vi "例4.3.vi"() -> ()   [LabVIEW 2018]
panel:
  out "MAX":dbl
  in  "y":dbl
  in  "x":dbl
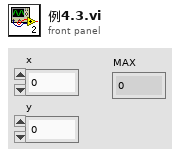
[diagram p1: front panel]
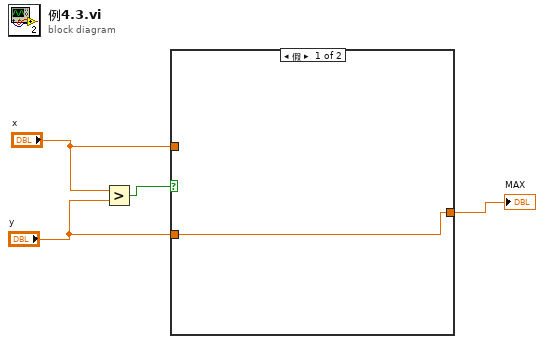
[diagram p0: block diagram]
diagram:
  n1 = Greater?(x="x", y="y") -> (0:w4:bool)
  n2 = case shown="假" w4 {
    tunnel: [w5 w6] -> w1
    tunnel: "x" -> [_ w6]
    tunnel: "y" -> [w5 _]
    frame False {
    }
    frame True {
    }
  }
  "MAX" <- w1
